vi "Test Sensing.vi"() -> ()   [LabVIEW 2019]
uses:
  <vilib>/myRIO/Instrument Drivers/Onboard IO/I2C/typedefs/I2C User Configuration.ctl
  <vilib>/myRIO/Instrument Drivers/Onboard IO/I2C/typedefs/I2C Transfer Rate.ctl
  <vilib>/myRIO/Instrument Drivers/Onboard IO/I2C/typedefs/I2C Reference.ctl
  <vilib>/myRIO/Common/Instrument Driver Framework/Utilities/typedefs/myRIO Generic Hardware Reference.ctl
  <vilib>/myRIO/Common/Instrument Driver Framework/Utilities/typedefs/Hardware Version Enum.ctl
  <vilib>/myRIO/Common/Instrument Driver Framework/Utilities/typedefs/myRIO v1.0 Reference.ctl
  <vilib>/myRIO/Common/Instrument Driver Framework/Utilities/typedefs/Generic FPGA Reference.ctl
  <vilib>/myRIO/Common/Instrument Driver Framework/myRIO v1.0/I2C/typedefs/I2C Channels Enum.ctl
  <vilib>/myRIO/Instrument Drivers/Onboard IO/I2C/typedefs/I2C Configuration.ctl
  <vilib>/userDefined/High Color/nirio_resource_hc.ctl
  <vilib>/Platform/TimedLoop/XDataNode/timing_clust.ctl
  <vilib>/Platform/TimedLoop/XDataNode/nitl_modes.ctl
  <vilib>/Platform/TimedLoop/XDataNode/wakeup.ctl
  <vilib>/myRIO/Common/Instrument Driver Framework/Utilities/vis/Is FPGA Ref Available.vi
  <vilib>/myRIO/Common/Instrument Driver Framework/myRIO v1.0/I2C/vis/myRIO v1.1 Open I2C.vi
  <vilib>/myRIO/Instrument Drivers/Onboard IO/I2C/vis/Configure.vi
  <vilib>/myRIO/Instrument Drivers/Onboard IO/I2C/vis/Write.vi
  <vilib>/myRIO/Instrument Drivers/Onboard IO/I2C/vis/Write Read.vi
  <vilib>/myRIO/Common/Instrument Driver Framework/Utilities/vis/Validate Channels.vi
  <vilib>/myRIO/Common/Instrument Driver Framework/myRIO v1.0/I2C/vis/myRIO v1.0 Reserve I2C.vi
  <vilib>/myRIO/Common/Instrument Driver Framework/myRIO v1.0/UART/vis/myRIO v1.0 Close UART.vi
  <vilib>/myRIO/Common/Instrument Driver Framework/myRIO v1.0/I2C/vis/myRIO v1.0 Build MUX Configuration I2C.vi
  <vilib>/myRIO/Common/Instrument Driver Framework/myRIO v1.0/Resource Manager/vis/myRIO v1.0 Reserve Channel List.vi
  <vilib>/myRIO/Common/Instrument Driver Framework/myRIO v1.0/Resource Manager/vis/myRIO v1.0 Create Configuration List.vi
  <vilib>/myRIO/Common/Instrument Driver Framework/myRIO v1.0/Resource Manager/vis/myRIO v1.0 Reserve Channel.vi
  <vilib>/myRIO/Common/Instrument Driver Framework/myRIO v1.0/Resource Manager/vis/myRIO v1.0 Unreserve Channel.vi
  <vilib>/myRIO/Common/Instrument Driver Framework/myRIO v1.0/Resource Manager/vis/myRIO v1.0 Build Mutex Name.vi
  <vilib>/Utility/VariantDataType/GetNumericInfo.vi
  <vilib>/Utility/error.llb/Error Cluster From Error Code.vi
  <vilib>/myRIO/Common/Instrument Driver Framework/myRIO v1.0/myRIO v1.1 Open.vi
  <vilib>/myRIO/Common/Instrument Driver Framework/Utilities/vis/IO Manager.vi
  <vilib>/myRIO/Common/Instrument Driver Framework/Utilities/vis/Configuration Manager.vi
  <vilib>/myRIO/Common/Instrument Driver Framework/myRIO v1.0/Resource Manager/vis/myRIO v1.0 Configure IO.vi
  <vilib>/myRIO/Common/Instrument Driver Framework/myRIO v1.0/myRIO v1.0 Close.vi
  <vilib>/myRIO/Common/Instrument Driver Framework/myRIO v1.0/I2C/vis/myRIO v1.0 Configure I2C.vi
  <vilib>/myRIO/Common/Instrument Driver Framework/myRIO v1.0/I2C/vis/myRIO v1.0 Write I2C.vi
  <vilib>/myRIO/Common/Instrument Driver Framework/myRIO v1.0/I2C/vis/myRIO v1.0 Read I2C.vi
  <vilib>/myRIO/Common/Instrument Driver Framework/Utilities/vis/FPGA Ref Manager.vi
  <vilib>/myRIO/Common/Instrument Driver Framework/myRIO v1.0/myRIO v1.0 Reset FPGA.vi
  <vilib>/myRIO/Common/Instrument Driver Framework/myRIO v1.0/IRQ/vis/myRIO v1.0 IRQ Info FGV.vi
  <vilib>/myRIO/Common/Instrument Driver Framework/myRIO v1.0/IRQ/vis/myRIO v1.0 Timer IRQ Info FGV.vi
  <vilib>/myRIO/Common/Instrument Driver Framework/myRIO v1.0/IRQ/vis/myRIO v1.0 ISR Agent.vi
  <vilib>/myRIO/Instrument Drivers/Utilities/vis/Reset Index.vi
  <vilib>/myRIO/Common/Instrument Driver Framework/myRIO v1.0/Resource Manager/vis/myRIO v1.0 Block Write Resource Manager.vi
  <vilib>/myRIO/Express VI/Onboard IO/I2C/I2C Express VI.xnode
  <vilib>/myRIO/Instrument Drivers/Onboard IO/I2C/vis/myRIO I2C Open.xnode
  <vilib>/platform/TimedLoop/XDataNode/XDataNode.xnode
  <vilib>/myRIO/Instrument Drivers/Onboard IO/I2C/I2C.lvlib
  <vilib>/Platform/TimedLoop/XDataNode/XDNodeRunTimeDep.lvlib
  <vilib>/myRIO/Instrument Drivers/Utilities/Utilities.lvlib
panel:
  out "Y 7":i16
  out "Z 7":i16
  out "Magnetic field [G] 72-1 2":cluster{dbl, dbl, dbl}(graph) caption="Waveform Chart"
  out "Z_mag 7":dbl
  out "Y_mag 7":dbl
  out "X_mag 7":dbl
  out "X 7":i16
  out "Y 6":i16
  out "Z 6":i16
  out "Magnetic field [G] 72-1":cluster{dbl, dbl, dbl}(graph) caption="Waveform Chart"
  out "Z_mag 6":dbl
  out "Y_mag 6":dbl
  out "X_mag 6":dbl
  out "X 6":i16
  in  "stop":bool
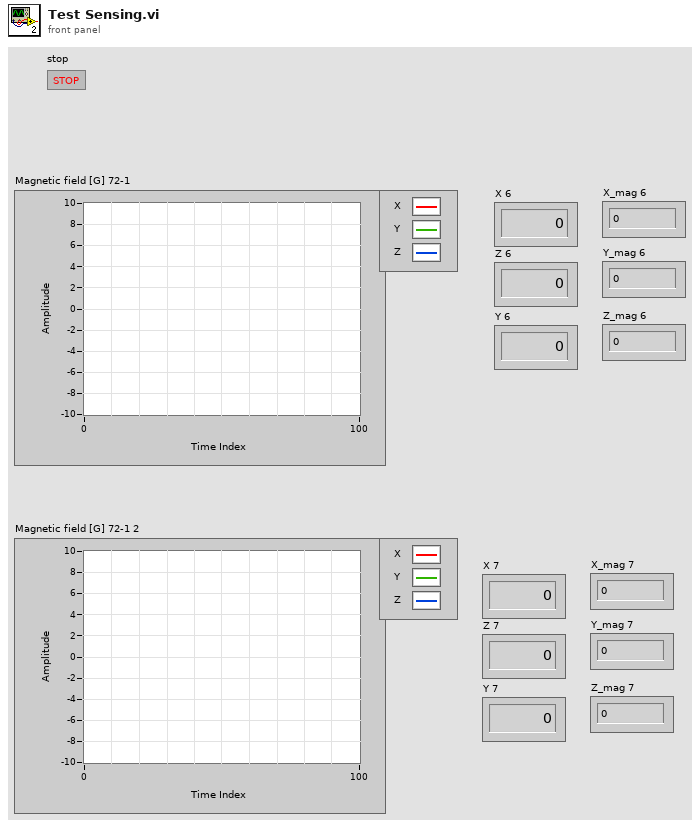
[diagram p1: front panel]
types:
  T1 = typedef "I2C.lvlib/I2C Reference.ctl" = cluster{"myRIO Reference":T2, "I2C Channels Enum":T6, "I2C Configuration":T7}
  T2 = typedef "myRIO Generic Hardware Reference.ctl" = cluster{"myRIO Model":T3, "myRIO Hardware Reference":T4}
  T3 = typedef "Hardware Version Enum.ctl" = enum16{"Unknown", "myRIO-1900", "myRIO-1950", "roboRIO", "NI ELVIS RIO CM", "ELVIS III"}
  T4 = typedef "myRIO v1.0 Reference.ctl" = cluster{"Generic FPGA Reference":T5, "Allow multiple opens":bool}
  T5 = typedef "Generic FPGA Reference.ctl" = refnum<k20>
  T6 = typedef "I2C Channels Enum.ctl" = enum16{"Not Connected", "A/I2C", "B/I2C", "I2C/I2C"}
  T7 = typedef "I2C.lvlib/I2C Configuration.ctl" = cluster{"I2C Transfer Rate":T8}
  T8 = typedef "I2C.lvlib/I2C Transfer Rate.ctl" = enum16{"Standard mode (100 kbps)", "Fast mode (400 kbps)"}
  T9 = typedef "I2C.lvlib/I2C User Configuration.ctl" = cluster{"I2C Transfer Rate":T8}
  T10 = typedef "nirio_resource_hc.ctl" = tag
  T11 = typedef "XDNodeRunTimeDep.lvlib/timing_clust.ctl" = cluster{"Expected End [f-1]":u64, "Actual End [f-1]":u64, "Finished Late? [f-1]":bool, "Expected End [i-1]":u64, "Actual End [i-1]":u64, "Finished Late? [i-1]":bool, "Expected Start [i]":u64, "Actual Start [i]":u64, "Expected Start [f]":u64, "Actual Start [f]":u64, "Source Name":string, "Structure Name":string, "Period":i64, "Deadline":i64, "Offset":i64, "Start":i64, "Priority":i32, "Timeout":i32, "Mode":T12, "Wakeup Reason":T13, "Error":errorcluster, "Source Type":string, "Secondary Source Type":string, "Global End Time":u64, "Global Start Time":u64, "Frame Duration":u64, "Iteration Duration":u64, "Assigned CPU":i32, "I/O Scan Engine Mode":u32}
  T12 = typedef "XDNodeRunTimeDep.lvlib/nitl_modes.ctl" = enum32{"No Change", "Process missed periods, maintain original phase", "Discard missed periods, maintain original phase", "Process missed periods, ignore original phase", "Discard missed periods, ignore original phase"}
  T13 = typedef "XDNodeRunTimeDep.lvlib/wakeup.ctl" = enum32{"Normal", "Aborted", "Asynchronous wakeup", "Timing source error", "Timed loop error", "Timeout"}
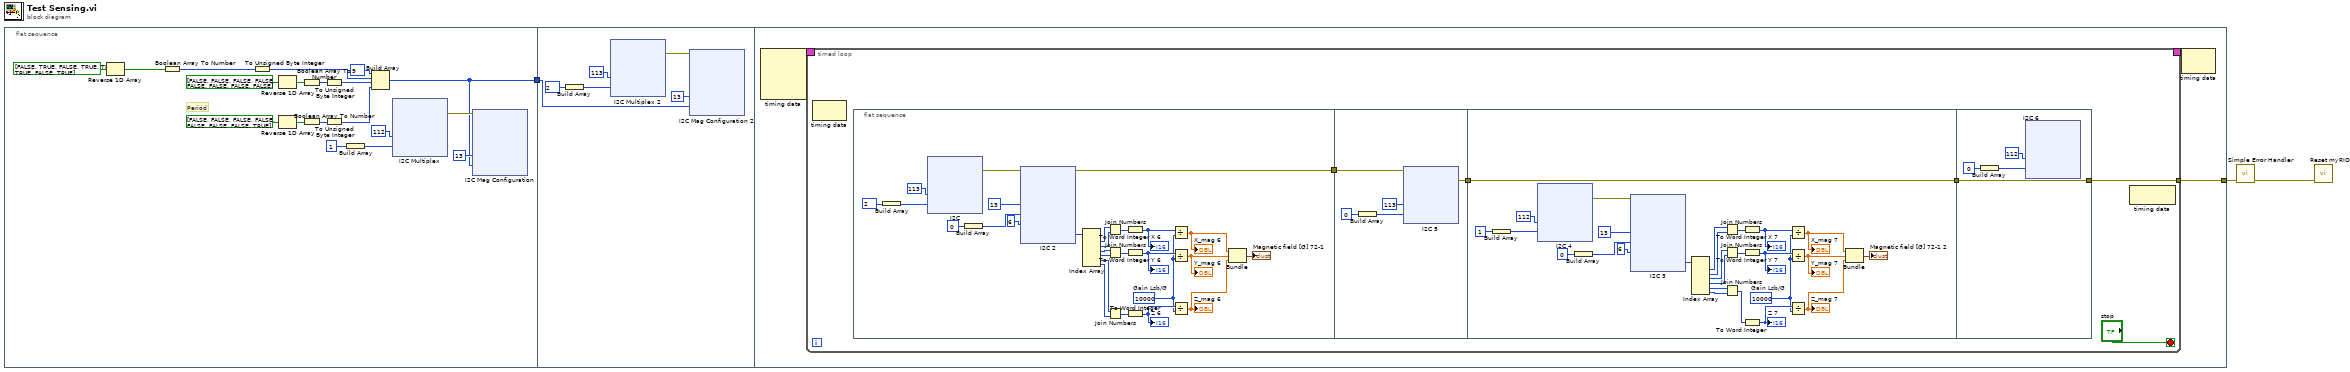
[diagram p0: block diagram]
diagram:
  n1 = flat-sequence {
    tunnel: [w6] -> w1
    tunnel: w1 -> [w101]
    tunnel: [w181] -> w2
    frame #0 {
      # "Period"
      n2 = Reverse 1D Array(array=bool[] [FALSE, TRUE, FALSE, TRUE, TRUE, TRUE, FALSE, TRUE]) -> (reversed array=w13:bool[])
      n3 = Boolean Array To Number(Boolean array=w13) -> (number=w16:u32)
      n4 = To Unsigned Byte Integer(number=w16) -> (unsigned 8bit integer=w19:u8)
      n5 = Reverse 1D Array(array=bool[] [FALSE, FALSE, FALSE, FALSE, FALSE, FALSE, FALSE, FALSE]) -> (reversed array=w14:bool[])
      n6 = Reverse 1D Array(array=bool[] [FALSE, FALSE, FALSE, FALSE, FALSE, FALSE, FALSE, TRUE]) -> (reversed array=w15:bool[])
      n7 = Boolean Array To Number(Boolean array=w14) -> (number=w17:u32)
      n8 = Boolean Array To Number(Boolean array=w15) -> (number=w18:u32)
      n9 = To Unsigned Byte Integer(number=w17) -> (unsigned 8bit integer=w20:u8)
      n10 = To Unsigned Byte Integer(number=w18) -> (unsigned 8bit integer=w21:u8)
      n11 = Build Array(u8 1) -> (w4:u8[])
      n12 = Build Array "Build Array"(u8 9 ("address"), w19, w20, w21) -> (w6:u8[])
      n13 = xnode "I2C Multiplex"("Slave Address (7-bit)"=u8 112, "Bytes to Write"=w4) -> ("error out"=w22:errorcluster)  [unwired: 1 in]
      n14 = xnode "I2C Mag Configuration"("Slave Address (7-bit)"=u8 13, "Bytes to Write"=w6, "error in (no error)"=w22) -> ()  [unwired: 1 out]
    }
    frame #1 {
      n15 = Build Array(u8 2) -> (w99:u8[])
      n16 = xnode "I2C Multiplex 2"("Slave Address (7-bit)"=u8 113, "Bytes to Write"=w99) -> ("error out"=w104:errorcluster)  [unwired: 1 in]
      n17 = xnode "I2C Mag Configuration 2"("Slave Address (7-bit)"=u8 13, "Bytes to Write"=w101, "error in (no error)"=w104) -> ()  [unwired: 1 out]
    }
    frame #2 {
      n18 = node-c288() -> (w183:T11)  [unwired: 4 in]
      n19 = timed-loop {
        timing: w183 -> [_]
        timing-out: [_] -> w182
        tunnel: [w186] -> w181
        stop <- "stop" stop-if-true
        n20 = node-c288() -> ()  [unwired: 1 in, 1 out]
        n21 = flat-sequence {
          tunnel: [w192] -> w187
          tunnel: w187 -> [w295]
          tunnel: [w294] -> w185
          tunnel: w185 -> [w363]
          tunnel: [w363] -> w184
          tunnel: [w445] -> w186
          tunnel: w184 -> [w445]
          frame #0 {
            w197 = i16 10000  # Gain Lsb/G
            n22 = Build Array(u8 2) -> (w189:u8[])
            n23 = xnode "I2C"("Slave Address (7-bit)"=u8 113, "Bytes to Write"=w189) -> ("error out"=w193:errorcluster)  [unwired: 1 in]
            n24 = Build Array(u8 0) -> (w198:u8[])
            n25 = xnode "I2C 2"("Slave Address (7-bit)"=u8 13, "Bytes to Write"=w198, "Byte Count"=u32 6, "error in (no error)"=w193) -> ("Bytes Read"=w208:u8[], "error out"=w192:errorcluster)
            n26 = Index Array(array=w208) -> (element #1=w207:u8, element #2=w206:u8, element #3=w205:u8, element #4=w204:u8, element #5=w203:u8, element #6=w202:u8)  [unwired: 6 in]
            n27 = Join Numbers(hi=w207, lo=w206) -> ((hi.lo)=w201:u16)
            n28 = Join Numbers(hi=w205, lo=w204) -> ((hi.lo)=w200:u16)
            n29 = Join Numbers(hi=w203, lo=w202) -> ((hi.lo)=w199:u16)
            n30 = To Word Integer(number=w201) -> (16bit integer=w213:i16)
            "X 6" <- w213
            n31 = To Word Integer(number=w200) -> (16bit integer=w215:i16)
            "Y 6" <- w215
            n32 = To Word Integer(number=w199) -> (16bit integer=w214:i16)
            "Z 6" <- w214
            n33 = Divide(x=w213, y=w197) -> (x/y=w209:dbl)
            "X_mag 6" <- w209
            n34 = Divide(x=w215, y=w197) -> (x/y=w210:dbl)
            "Y_mag 6" <- w210
            n35 = Divide(x=w214, y=w197) -> (x/y=w211:dbl)
            "Z_mag 6" <- w211
            n36 = Bundle(w209, w210, w211) -> (→"Magnetic field [G] 72-1":cluster{dbl, dbl, dbl})  [unwired: 1 in]
          }
          frame #1 {
            n37 = Build Array(u8 0) -> (w296:u8[])
            n38 = xnode "I2C 5"("Slave Address (7-bit)"=u8 113, "Bytes to Write"=w296, "error in (no error)"=w295) -> ("error out"=w294:errorcluster)
          }
          frame #2 {
            w344 = i16 10000  # Gain Lsb/G
            n39 = Build Array(u8 1) -> (w338:u8[])
            n40 = xnode "I2C 4"("Slave Address (7-bit)"=u8 112, "Bytes to Write"=w338) -> ("error out"=w341:errorcluster)  [unwired: 1 in]
            n41 = Build Array(u8 0) -> (w345:u8[])
            n42 = xnode "I2C 3"("Slave Address (7-bit)"=u8 13, "Bytes to Write"=w345, "Byte Count"=u32 6, "error in (no error)"=w341) -> ("Bytes Read"=w355:u8[])  [unwired: 1 out]
            n43 = Index Array(array=w355) -> (element #1=w354:u8, element #2=w353:u8, element #3=w352:u8, element #4=w351:u8, element #5=w350:u8, element #6=w349:u8)  [unwired: 6 in]
            n44 = Join Numbers(hi=w354, lo=w353) -> ((hi.lo)=w348:u16)
            n45 = Join Numbers(hi=w352, lo=w351) -> ((hi.lo)=w347:u16)
            n46 = Join Numbers(hi=w350, lo=w349) -> ((hi.lo)=w346:u16)
            n47 = To Word Integer(number=w348) -> (16bit integer=w360:i16)
            "X 7" <- w360
            n48 = To Word Integer(number=w347) -> (16bit integer=w362:i16)
            "Y 7" <- w362
            n49 = To Word Integer(number=w346) -> (16bit integer=w361:i16)
            "Z 7" <- w361
            n50 = Divide(x=w360, y=w344) -> (x/y=w356:dbl)
            "X_mag 7" <- w356
            n51 = Divide(x=w362, y=w344) -> (x/y=w357:dbl)
            "Y_mag 7" <- w357
            n52 = Divide(x=w361, y=w344) -> (x/y=w358:dbl)
            "Z_mag 7" <- w358
            n53 = Bundle(w356, w357, w358) -> (→"Magnetic field [G] 72-1 2":cluster{dbl, dbl, dbl})  [unwired: 1 in]
          }
          frame #3 {
            n54 = Build Array(u8 0) -> (w442:u8[])
            n55 = xnode "I2C 6"("Slave Address (7-bit)"=u8 112, "Bytes to Write"=w442) -> ()  [unwired: 1 in, 1 out]
          }
        }
        n56 = node-c288() -> ()  [unwired: 1 in, 1 out]
      }
      n57 = node-c288(w182) -> ()  [unwired: 1 out]
    }
  }
  n58 = call <vilib>:"Simple Error Handler.vi"("error in (no error)"=w2) -> ("error out"=w3:errorcluster)  [unwired: 4 in, 4 out]
  n59 = call <vilib>:"Reset myRIO.vi"("error in (no error)"=w3) -> ()  [unwired: 10 in, 1 out]
